vi "BeadCooler(SubVI).vi"(0 "Enum":T1(ring), 1 "Input":i16, 2 "Setpoint":fxp<+/-,16,16>, 5 "low pass coefficients":i32[](array[numeric])=[0, 0, 0, 0, 0, 0], 7 "dg":fxp<+/-,32,16>, 9 "pg":fxp<+/-,32,16>, 11 "Reset after samps":u16, 12 "Dc offset":fxp<+/-,32,16>, 13 "Upper lim":fxp<+/-,32,16>, 14 "Lower lim":fxp<+/-,32,16>, 15 "Num samps to reset":u16) -> (4 "Filtered Input":fxp<+/-,20,20>, 6 "Output":fxp<+/-,32,16>, 10 "derivative":fxp<+/-,22,22>)   [LabVIEW 2012]
uses:
  <vilib>/rvi/Analysis/measure/butterworth/XNode/niFpgaButterworthFilter.xnode
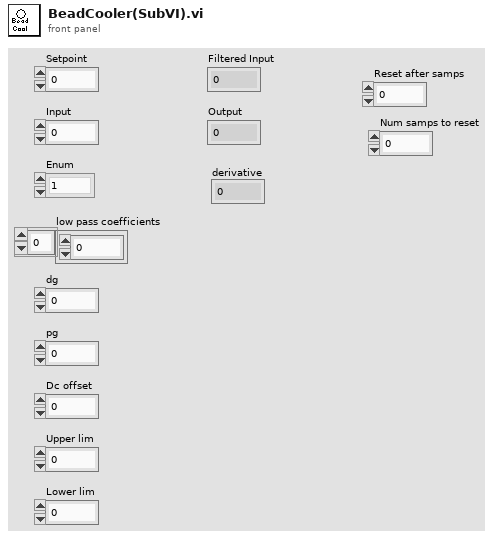
[diagram p1: front panel]
types:
  T1 = enum16{"1", "2", "4", "8", "16", "32", "64", "128", "256", "512"}
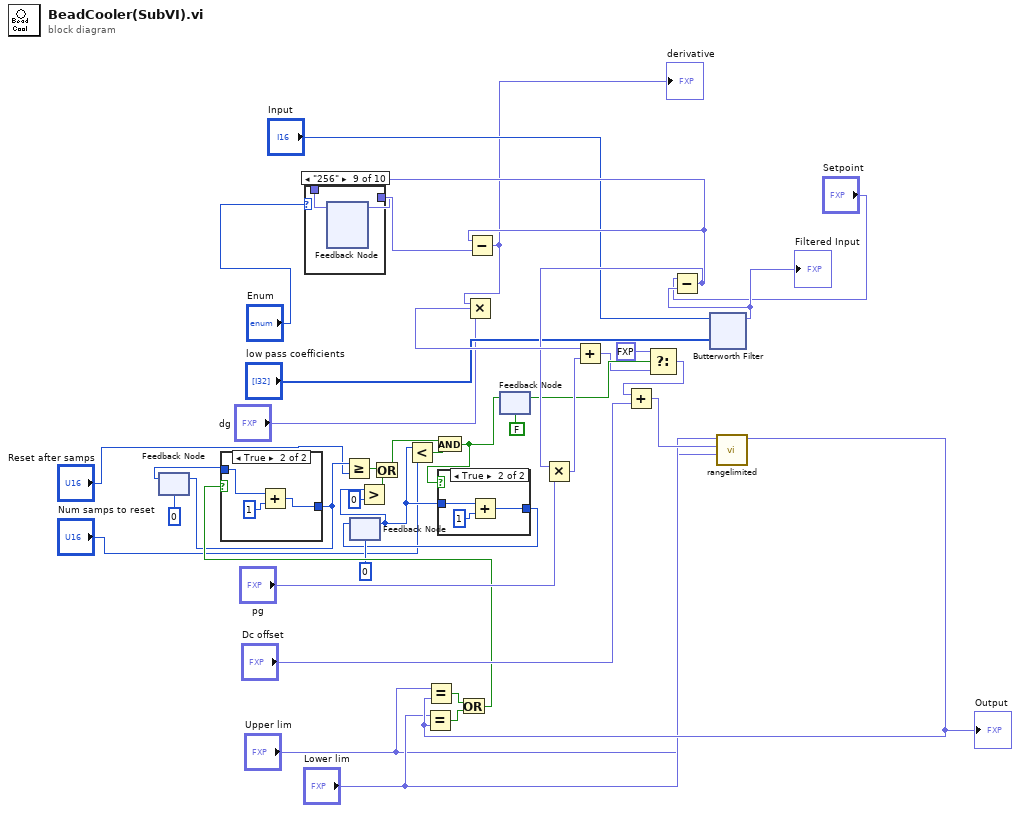
[diagram p0: block diagram]
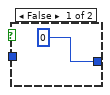
[diagram p2: hidden frame]
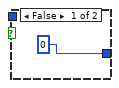
[diagram p3: hidden frame]
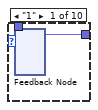
[diagram p4: hidden frame]
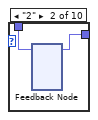
[diagram p5: hidden frame]
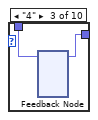
[diagram p6: hidden frame]
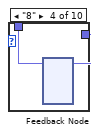
[diagram p7: hidden frame]
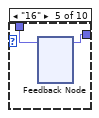
[diagram p8: hidden frame]
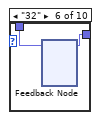
[diagram p9: hidden frame]
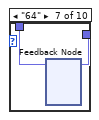
[diagram p10: hidden frame]
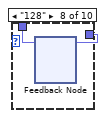
[diagram p11: hidden frame]
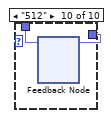
[diagram p12: hidden frame]
diagram:
  n1 = feedback #1(u16 0 ("t")) -> (w17:u16)
  n2 = feedback #2(u16 0 ("t")) -> (w7:u16)
  n3 = Greater?(x=w7, y=u16 0) -> (0:w12:bool)
  n4 = Less?(x=w7, y="Num samps to reset") -> (x < y?=w8:bool)
  n5 = feedback #3(FALSE) -> (w4:bool)
  n6 = xnode "Butterworth Filter"("input data"="Input", "scaled coefficients"="low pass coefficients") -> ("output data"=w36:fxp<+/-,20,20>)  [unwired: 1 in]
  "Filtered Input" <- w36
  n7 = Subtract(x="Setpoint", y=w36) -> (x-y=w34:fxp<+/-,21,21>)
  n8 = case shown="\"256\"" "Enum" {
    tunnel: [w41 w42 w44 w46 w48 w50 w52 w54 w56 w58] -> w27
    tunnel: w34 -> [w40 w43 w45 w47 w49 w51 w53 w55 w57 w59]
    frame "1" {
      n9 = feedback #4() -> (w41:fxp<+/-,21,21>)  [unwired: 1 in]
      n10 = feedback-in #4(w40) -> ()
    }
    frame "2" {
      n11 = feedback #5() -> (w42:fxp<+/-,21,21>)  [unwired: 1 in]
      n12 = feedback-in #5(w43) -> ()
    }
    frame "4" {
      n13 = feedback #6() -> (w44:fxp<+/-,21,21>)  [unwired: 1 in]
      n14 = feedback-in #6(w45) -> ()
    }
    frame "8" {
      n15 = feedback #7() -> (w46:fxp<+/-,21,21>)  [unwired: 1 in]
      n16 = feedback-in #7(w47) -> ()
    }
    frame "16" {
      n17 = feedback #8() -> (w48:fxp<+/-,21,21>)  [unwired: 1 in]
      n18 = feedback-in #8(w49) -> ()
    }
    frame "32" {
      n19 = feedback #9() -> (w50:fxp<+/-,21,21>)  [unwired: 1 in]
      n20 = feedback-in #9(w51) -> ()
    }
    frame "64" {
      n21 = feedback #10() -> (w52:fxp<+/-,21,21>)  [unwired: 1 in]
      n22 = feedback-in #10(w53) -> ()
    }
    frame "128" {
      n23 = feedback #11() -> (w54:fxp<+/-,21,21>)  [unwired: 1 in]
      n24 = feedback-in #11(w55) -> ()
    }
    frame "256" {
      n25 = feedback #12() -> (w56:fxp<+/-,21,21>)  [unwired: 1 in]
      n26 = feedback-in #12(w57) -> ()
    }
    frame "512" {
      n27 = feedback #13() -> (w58:fxp<+/-,21,21>)  [unwired: 1 in]
      n28 = feedback-in #13(w59) -> ()
    }
  }
  n29 = Subtract(x=w34, y=w27) -> (x-y=w28:fxp<+/-,22,22>)
  "derivative" <- w28
  n30 = Multiply(x=w28, y="dg") -> (x*y=w39:fxp<+/-,53,37>)
  n31 = Multiply(x=w34, y="pg") -> (x*y=w35:fxp<+/-,52,36>)
  n32 = Add(x=w39, y=w35) -> (x+y=w2:fxp<+/-,53,37>)
  n33 = Select(t=fxp<+/-,32,16> 0.0, s=w4, f=w2) -> (s? t:f=w19:fxp<+/-,53,37>)
  n34 = Add(x=w19, y="Dc offset") -> (x+y=w38:fxp<+/-,53,37>)
  n35 = call "rangelimited.vi"("Upper lim"="Upper lim", "Input"=w38, "Lower lim"="Lower lim") -> ("Output"=w25:fxp<+/-,32,16>)  [unwired: 8 in]
  "Output" <- w25
  n36 = Equal?(x="Lower lim", y=w25) -> (x = y?=w21:bool)
  n37 = Equal?(x="Upper lim", y=w25) -> (x = y?=w22:bool)
  n38 = Or(x=w22, y=w21) -> (x .or. y?=w20:bool)
  n39 = case shown="True" w20 {
    tunnel: [u16 0 ("t") w62] -> w16
    tunnel: w17 -> [_ w61]
    frame False {
    }
    frame True {
      n40 = Add(x=w61, y=u16 1 ("t")) -> (x+y=w62:u16)
    }
  }
  n41 = feedback-in #1(w16) -> ()
  n42 = Greater Or Equal?(x=w16, y="Reset after samps") -> (x >= y?=w13:bool)
  n43 = Or(x=w13, y=w12) -> (x .or. y?=w9:bool)
  n44 = And(x=w9, y=w8) -> (x .and. y?=w5:bool)
  n45 = case shown="True" w5 {
    tunnel: [u16 0 ("t") w66] -> w11
    tunnel: w7 -> [_ w65]
    frame False {
    }
    frame True {
      n46 = Add(x=w65, y=u16 1 ("t")) -> (x+y=w66:u16)
    }
  }
  n47 = feedback-in #2(w11) -> ()
  n48 = feedback-in #3(w5) -> ()
